vi "LWConexCC_Open.vi"(6 "Instrument Key IN":string) -> (0 "error out":errorcluster, 1 "return code":i32, 2 "Instrument Key OUT":string, 3 "ConexCC Reference":refnum<k24>)   [LabVIEW 2015]
uses:
  Newport.CONEXCC.CommandInterface
panel:
  out "InstrumentKeys":string[](array[string])
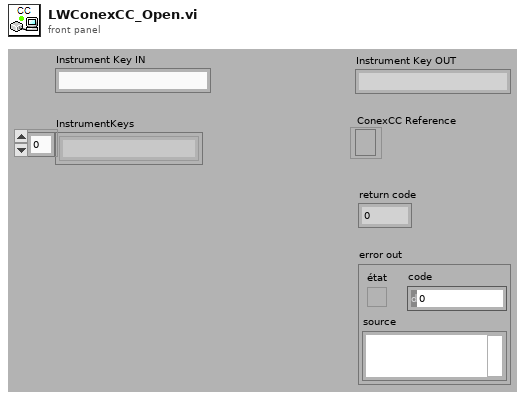
[diagram p1: front panel]
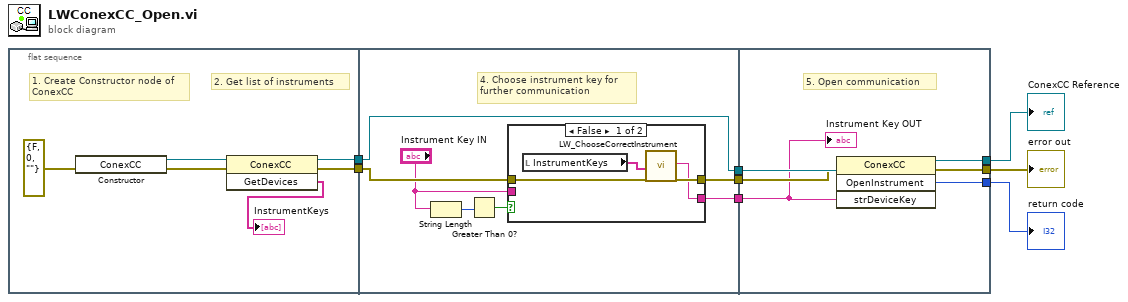
[diagram p0: block diagram]
diagram:
  n1 = flat-sequence {
    tunnel: [w12] -> w2
    tunnel: [w11] -> w1
    tunnel: w2 -> [w15]
    tunnel: w1 -> [w19]
    tunnel: [w15] -> w8
    tunnel: [w18] -> w7
    tunnel: [w16] -> w6
    tunnel: w8 -> [w33]
    tunnel: w7 -> [w32]
    tunnel: w6 -> [w31]
    tunnel: [w30] -> w5
    tunnel: [w29] -> w4
    tunnel: [w28] -> w3
    frame #0 {
      # "1. Create Constructor node of \nConexCC"
      # "2. Get list of instruments"
      n2 = constructor class="ConexCC"(error in=errorcluster {"status"=FALSE, "code"=0, "source"=""} ("entrée d'erreur (pas d'erreur)")) -> (reference out=w14:refnum<k24>, error out=w13:errorcluster)  [unwired: 2 in, 1 out]
      n3 = invoke class="ConexCC" method="GetDevices"(reference=w14, error in=w13) -> (reference out=w12:refnum<k24>, error out=w11:errorcluster, "GetDevices"=→"InstrumentKeys":string[])  [unwired: 1 in]
    }
    frame #1 {
      # "4. Choose instrument key for \nfurther communication"
      n4 = String Length(string="Instrument Key IN") -> (length=w21:i32)
      n5 = Greater Than 0?(x=w21) -> (x > 0?=w20:bool)
      n6 = case shown="False" w20 {
        tunnel: w19 -> [w25 w27]
        tunnel: [w23 w27] -> w18
        tunnel: [w22 w26] -> w16
        tunnel: "Instrument Key IN" -> [_ w26]
        frame False {
          n7 = local read "InstrumentKeys"() -> (w24:string[])
          n8 = call "LW_ChooseCorrectInstrument.vi"("Instrument Keys"=w24, "error in (no error)"=w25) -> ("selected instrument key"=w22:string, "error out"=w23:errorcluster)  [unwired: 16 in]
        }
        frame True {
        }
      }
    }
    frame #2 {
      # "5. Open communication"
      n9 = invoke class="ConexCC" method="OpenInstrument"(reference=w33, error in=w32, "strDeviceKey"=w31) -> (reference out=w30:refnum<k24>, error out=w29:errorcluster, "OpenInstrument"=w28:i32)  [unwired: 1 in, 1 out]
      "Instrument Key OUT" <- w31
    }
  }
  "error out" <- w4
  "return code" <- w3
  "ConexCC Reference" <- w5
